vi "WPI_ADI_IMU_Reset.vi"(8 "error in":errorcluster, 11 "ADI IMU Interrupt DevRef":T1={"ADI IMU DevRef"={"DevStatus"={"status"=FALSE, "code"=0, "source"=""}, "Handle"=0, "SPI Bus"=enum."SPI On-Board, CS0", "Device Found"=FALSE, "Device Ready"=FALSE, "Yaw Axis"=enum."Z", "AHRS Algorithm"=enum."Complementary"}, "InterruptRef"={"DevStatus"={"status"=FALSE, "code"=0, "source"=""}, "InterruptIndex"=enum."0"}}) -> (0 "error out":errorcluster, 3 "ADI IMU Interrupt DevRef Out":T1={"ADI IMU DevRef"={"DevStatus"={"status"=FALSE, "code"=0, "source"=""}, "Handle"=0, "SPI Bus"=enum."SPI On-Board, CS0", "Device Found"=FALSE, "Device Ready"=FALSE, "Yaw Axis"=enum."Z", "AHRS Algorithm"=enum."Complementary"}, "InterruptRef"={"DevStatus"={"status"=FALSE, "code"=0, "source"=""}, "InterruptIndex"=enum."0"}})   [LabVIEW 2015, in "FRC ADI MXP IMU.lvlib"]
doc: "Resets the accumulated angles to zero in software. This VI does NOT electrically reset the ADI MXP IMU or reset the calibration."
uses:
  FRC ADI MXP IMU.lvlib
  WPI_AnalogDevicesIMUInterruptDevRef.ctl
  WPI_AnalogDevicesIMUDevRef.ctl
  <vilib>/Rock Robotics/SystemInterfaces/spilib/spi_bus.ctl
  <vilib>/Rock Robotics/WPI/Interrupt/WPI_InterruptRef.ctl
  <vilib>/Rock Robotics/SystemInterfaces/Interrupt/FPGA_InterruptIndex.ctl
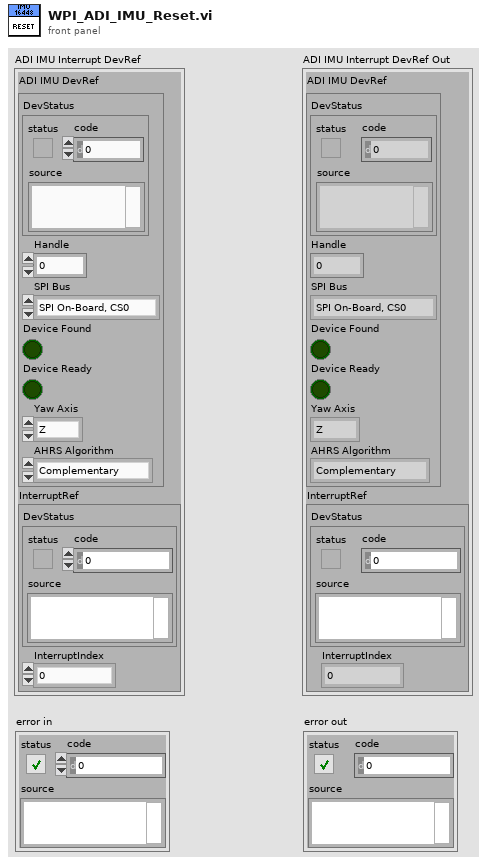
[diagram p1: front panel]
types:
  T1 = typedef "FRC ADI MXP IMU.lvlib/WPI_AnalogDevicesIMUInterruptDevRef.ctl" = cluster{"ADI IMU DevRef":T2, "InterruptRef":T4}
  T2 = typedef "FRC ADI MXP IMU.lvlib/WPI_AnalogDevicesIMUDevRef.ctl" = cluster{"DevStatus":errorcluster, "Handle":i32, "SPI Bus":T3, "Device Found":bool, "Device Ready":bool, "Yaw Axis":enum16{"X", "Y", "Z"}, "AHRS Algorithm":enum16{"Complementary", "Madgwick"}}
  T3 = typedef "spi_bus.ctl" = enum16{"SPI On-Board, CS0", "SPI On-Board, CS1", "SPI On-Board, CS2", "SPI On-Board, CS3", "SPI MXP", "Invalid"}
  T4 = typedef "WPI_InterruptRef.ctl" = cluster{"DevStatus":errorcluster, "InterruptIndex":T5}
  T5 = typedef "FPGA_InterruptIndex.ctl" = enum8{"0", "1", "2", "3", "4", "5", "6", "7", "Invalid"}
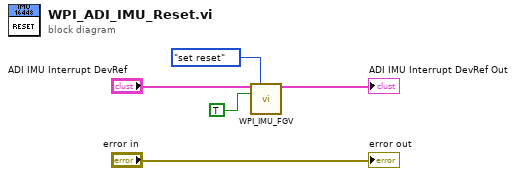
[diagram p0: block diagram]
diagram:
  n1 = call "WPI_IMU_FGV.vi"("ADI IMU Interrupt DevRef"="ADI IMU Interrupt DevRef", "Operation"=enum16{"set", "get", "set reset"}."set reset", "Reset"=TRUE) -> ("ADI IMU Interrupt DevRef Out"=→"ADI IMU Interrupt DevRef Out":T1)  [unwired: 6 in, 6 out]
  "error out" <- "error in"
